vi "Process.vi"(8 "error in (no error)":errorcluster, 10 "pound in":refnum<class "Pound.lvclass">, 11 "qbus in":refnum<class "Qbus.lvclass">) -> (0 "error out":errorcluster)   [LabVIEW 2017, in "TracePointSynchronizer.lvlib"]
doc: "This process runs in the Server Comm module to send tracepoint instances to NI InsightCM Server and inform the Tracelogger process when the list of enabled tracepoints changes."
uses:
  <vilib>/addons/InsightCM/Devices/Shared/Common/TracePointSynchronizer/TracePointSynchronizer.lvlib
  <vilib>/addons/Qbus/Qbus.lvclass
  <vilib>/NI/Software Watchdog/Pound/Pound.lvclass
  <vilib>/addons/InsightCM/Devices/Shared/Common/TracePointSynchronizer/controls/config.ctl
  <vilib>/addons/InsightCM/Devices/Shared/Common/ServerComm/controls/ConnectionStatus.ctl
  <vilib>/addons/InsightCM/MessageBus/Base/controls/Message.ctl
  <vilib>/addons/InsightCM/MessageBus/Base/controls/MessageHeader.ctl
  <vilib>/addons/InsightCM/MessageBus/Base/controls/KeyValuePair.ctl
  <vilib>/addons/TimerProcess/controls/taskType.ctl
  <vilib>/addons/InsightCM/MessageBus/MessageLibrary/TraceLogger/controls/TraceLoggerCommandRequestBody.ctl
  <vilib>/addons/TraceLogger/controls/TracepointConfig.ctl
  <vilib>/addons/TraceLogger/TraceLogger.lvlib
  <vilib>/NI/Software Watchdog/Watchdog/Watchdog.lvclass
  <vilib>/addons/InsightCM/Devices/Shared/Common/ServerComm/ServerComm.lvlib
  <vilib>/addons/InsightCM/Utilities/GlobalConfiguration/GlobalConfiguration.lvlib
  <vilib>/addons/TimerProcess/TimerProcess.lvlib
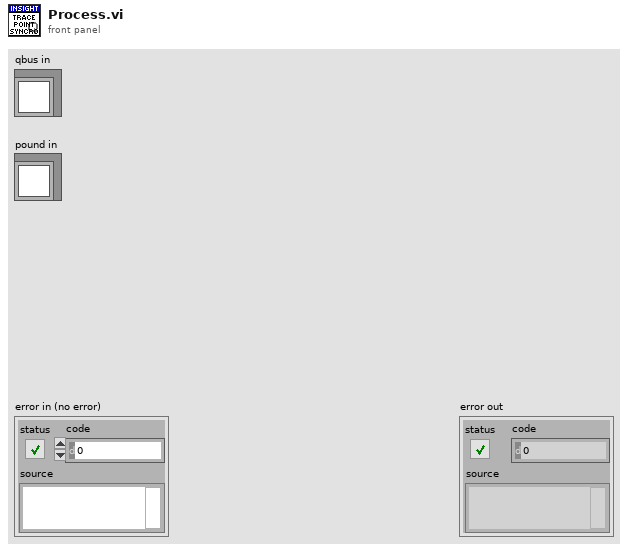
[diagram p1: front panel]
types:
  T1 = typedef "TracePointSynchronizer.lvlib/config.ctl" = cluster{"connection status":T2, "device name":string, "backlog messages":T3[], "log dir":path}
  T2 = typedef "ServerComm.lvlib/ConnectionStatus.ctl" = enum16{"Offline", "NotAuthorized", "Online"}
  T3 = typedef "Message.ctl" = cluster{"Header":T4, "Body":u8[]}
  T4 = typedef "MessageHeader.ctl" = cluster{"MessageName":string, "Timestamp":i64, "CorrelationId":string, "ContentType":string, "RoutingKey":string, "Properties":T5[]}
  T5 = typedef "KeyValuePair.ctl" = cluster{"Key":string, "Value":string}
  T6 = typedef "TimerProcess.lvlib/taskType.ctl" = enum16{"single", "repeat"}
  T7 = typedef "TraceLoggerCommandRequestBody.ctl" = cluster{"Arguments":string[]}
  T8 = typedef "TraceLogger.lvlib/TracepointConfig.ctl" = cluster{"name":string, "enabled":bool}
  T9 = typedef "R2_Device.ctl" = cluster{"Id":string, "Name":string, "DeviceType":string, "HardwareName":string, "IpAddress":string, "HardwareInfo":T5[], "ApplicationType":string, "ApplicationVersion":string, "EquipmentIds":string[], "ConfigurationVersion":string, "State":T10, "Properties":T5[], "DataGroups":T11[], "BurstModeTrigger":T15, "SensorGroups":T16[], "Endpoints":T17[]}
  T10 = typedef "DeviceState.ctl" = cluster{"Disabled":bool}
  T11 = typedef "R2_DataGroup.ctl" = cluster{"Name":string, "OperatingStates":T12[], "Properties":T5[], "EquipmentIds":string[], "AssetNodeId":string}
  T12 = typedef "OperatingState.ctl" = cluster{"Name":string, "Properties":T5[], "Triggers":T13[]}
  T13 = typedef "Trigger.ctl" = cluster{"Type":string, "Expression":string, "Conditions":T14[]}
  T14 = typedef "Condition.ctl" = cluster{"Source":string, "Type":string, "Operator":string, "CompareTo":string, "DwellSeconds":dbl}
  T15 = typedef "BurstModeTrigger.ctl" = cluster{"Trigger":T13, "SampleRate":string, "AcquisitionLength":string}
  T16 = typedef "DeviceSensorGroup.ctl" = cluster{"EquipId":string, "SensorGroupId":string}
  T17 = typedef "WirelessEndpoint.ctl" = cluster{"SerialNumber":string, "Properties":T5[], "Channels":T18[]}
  T18 = typedef "WirelessChannel.ctl" = cluster{"ChannelNumber":i32, "AssetId":string}
  T19 = typedef "TraceLoggerSnapshotBroadcastBody.ctl" = cluster{"Settings":T20[]}
  T20 = typedef "TracePointSetting.ctl" = cluster{"Name":string, "Enabled":bool, "Exceptions":string[]}
  T21 = typedef "TraceLogger.lvlib/LogTracepoint.ctl" = cluster{"tracepoint":string, "log string":string}
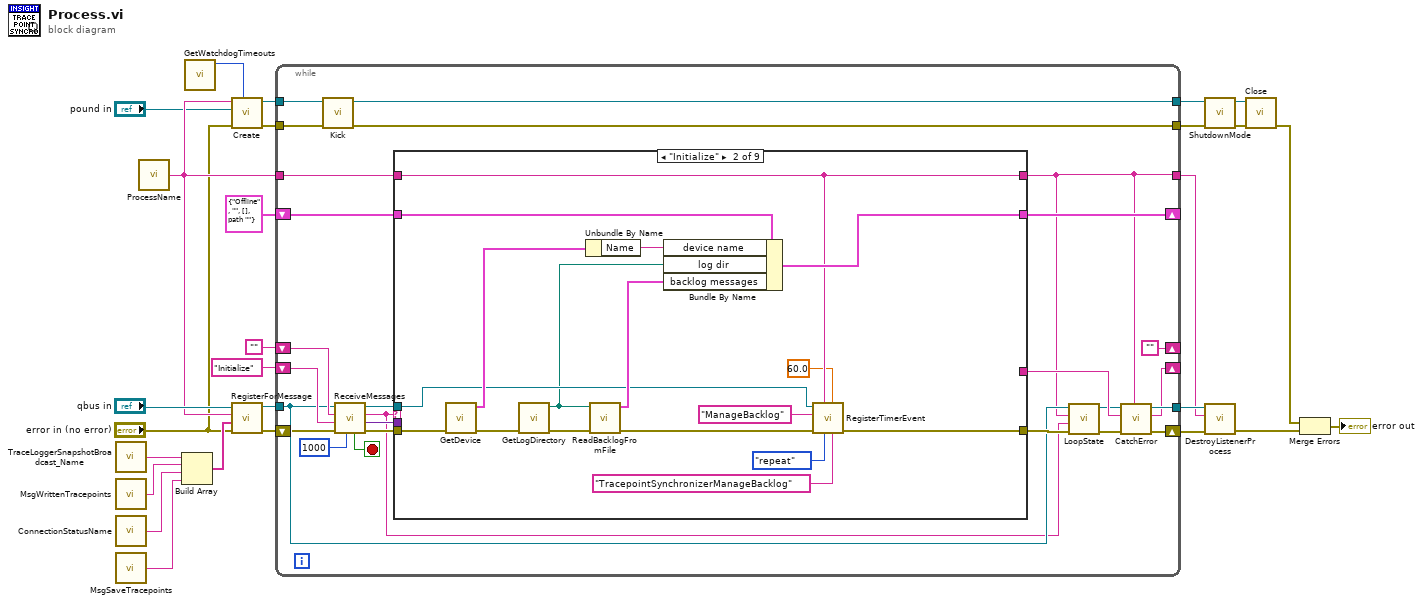
[diagram p0: block diagram]
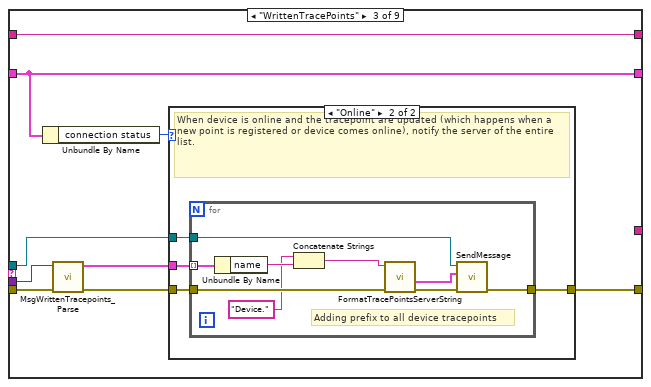
[diagram p3: hidden frame]
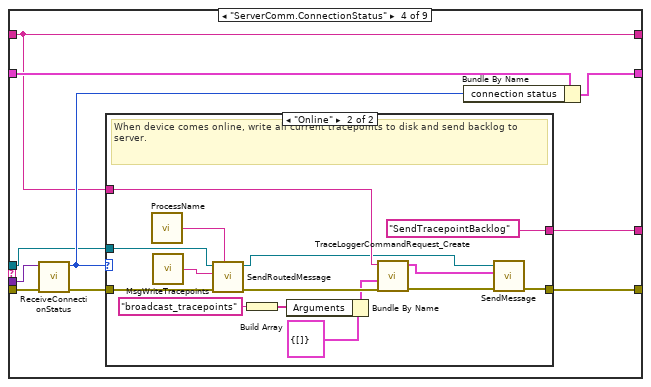
[diagram p5: hidden frame]
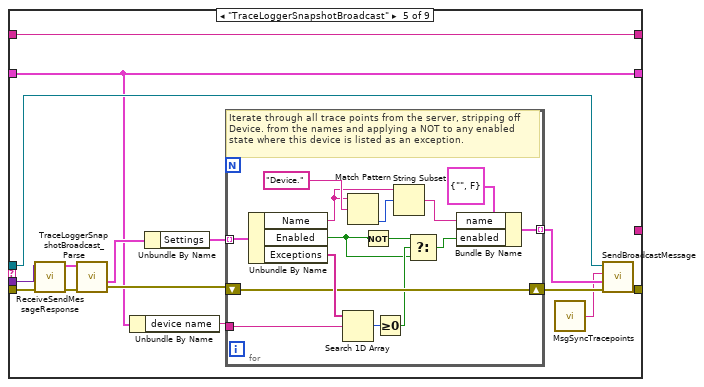
[diagram p7: hidden frame]
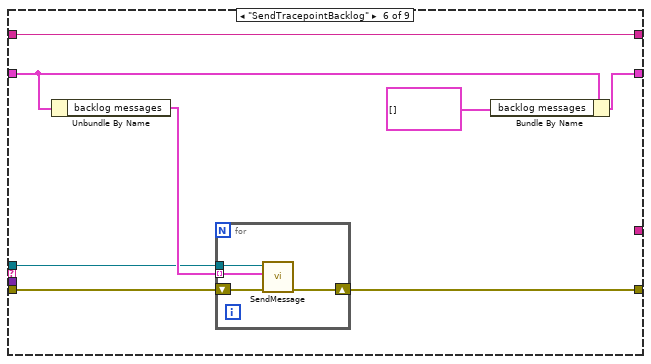
[diagram p8: hidden frame]
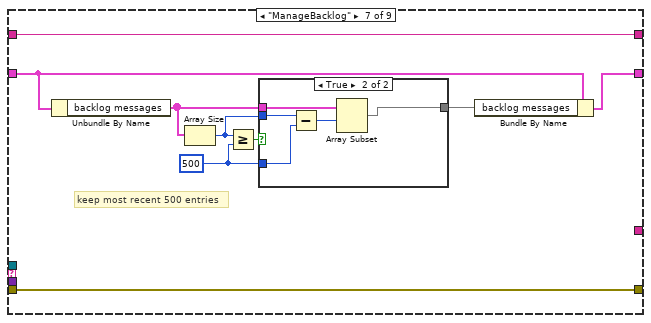
[diagram p9: hidden frame]
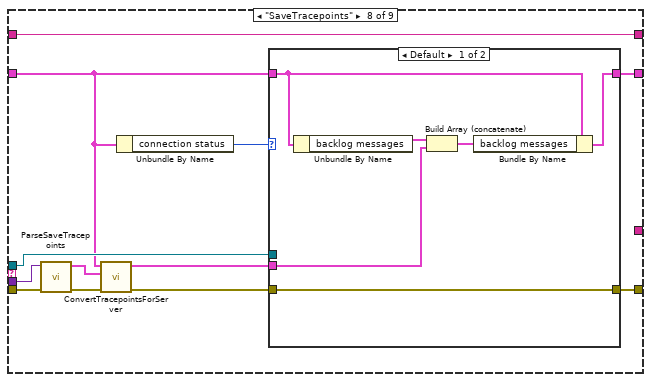
[diagram p11: hidden frame]
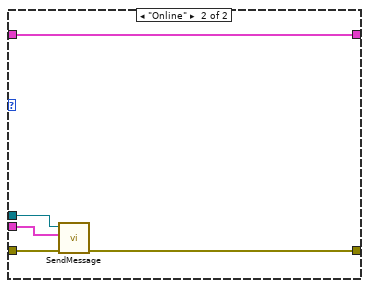
[diagram p12: hidden frame]
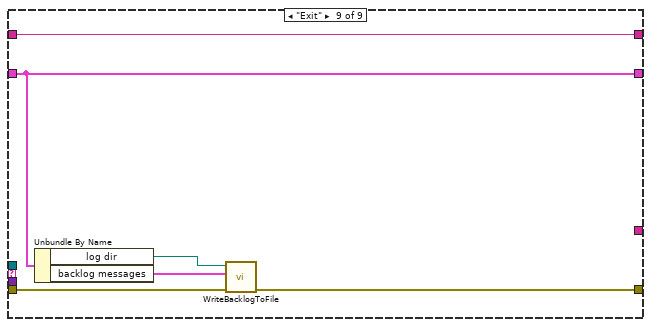
[diagram p13: hidden frame]
diagram:
  n1 = call <vilib>:"TraceLoggerSnapshotBroadcast_Name.vi"() -> ("MessageName"=w5:string)  [unwired: 5 in]
  n2 = call <vilib>:"MsgWrittenTracepoints.vi"() -> ("message name"=w4:string)  [unwired: 5 in]
  n3 = call <vilib>:"ConnectionStatusName.vi"() -> ("message name"=w3:string)  [unwired: 5 in]
  n4 = call <vilib>:"MsgSaveTracepoints.vi"() -> ("message name"=w2:string)  [unwired: 5 in]
  n5 = call <vilib>:"ProcessName.vi"() -> ("ProcessName"=w17:string)  [unwired: 5 in]
  n6 = Build Array(w5, w4, w3, w2) -> (w18:string[])
  n7 = call <vilib>:"GetWatchdogTimeouts.vi"() -> ("software timeout"=w1:u32)  [unwired: 10 in, 1 out]
  n8 = call <vilib>:"Create.vi"("Execution Timeout (ms)"=w1, "error in (no error)"="error in (no error)", "Pound"="pound in", "Name"=w17) -> ("error out"=w11:errorcluster, "Watchdog"=w16:refnum<data-value>)  [unwired: 6 in]
  n9 = call <vilib>:"RegisterForMessage.vi"("error in (no error)"="error in (no error)", "message names"=w18, "process name"=w17, "Qbus in"="qbus in") -> ("error in (no error)"=w26:errorcluster, "Qbus out"=w25:refnum<class "Qbus.lvclass">)  [unwired: 6 in]
  n10 = while {
    shift-right: [""] -> _
    shift-left: "" -> [w52]
    tunnel: w25 -> [w39]
    tunnel: w17 -> [w40]
    tunnel: [w43] -> w23
    tunnel: [w30] -> w22
    shift-right: [w42] -> _
    shift-left: "Initialize" -> [w47]
    shift-right: [w45] -> _
    shift-left: T1 {"connection status"=enum."Offline", "device name"="", "backlog messages"=[], "log dir"=path ""} ("config") -> [w46]
    tunnel: w16 -> [w38]
    tunnel: [w37] -> w13
    tunnel: w11 -> [w36]
    tunnel: [w34] -> w10
    shift-right: [w44] -> w24
    shift-left: w26 -> [w35]
    stop <- w53 stop-if-true
    n11 = call <vilib>:"Kick.vi"("error in (no error)"=w36, "Watchdog"=w38) -> ("error out"=w34:errorcluster, "Watchdog"=w37:refnum<data-value>)  [unwired: 8 in]
    n12 = call <vilib>:"ReceiveMessages.vi"("timeout(1000)"=1000 ("timeout(100)"), "error in (no error)"=w35, "priority action"=w47, "default action"=w52, "qbus in"=w39) -> ("error out"=w51:errorcluster, "message value"=w48:variant, "action"=w33:string, "qbus out"=w49:refnum<class "Qbus.lvclass">, "exit"=w53:bool)  [unwired: 2 in]
    n13 = case shown="\"Initialize\"" w33 {
      tunnel: w51 -> [w56 w73 w82 w106 w130 w156 w171 w191 w207]
      tunnel: w49 -> [_ w61 w79 w99 w133 w157 _ w187 _]
      tunnel: [w56 w60 w78 w101 w135 w155 w171 w186 w206] -> w41
      tunnel: w48 -> [_ _ w81 w105 w131 _ _ w190 _]
      tunnel: w46 -> [w55 w70 w80 w104 w125 w160 w173 w182 w208]
      tunnel: [w55 w69 w80 w103 w125 w159 w172 w181 w208] -> w45
      tunnel: w40 -> [w54 w63 w75 w97 w123 w153 w165 w180 w203]
      tunnel: [_ _ _ w98 _ _ _ _ _] -> w32
      tunnel: [w54 w63 w75 w97 w123 w153 w165 w180 w203] -> w30
      frame "", Default {
      }
      frame "Initialize" {
        n14 = call <vilib>:"GetDevice.vi"("error in (no error)"=w73) -> ("error out"=w59:errorcluster, "device configuration"=w72:T9)  [unwired: 8 in, 1 out]
        n15 = call <vilib>:"GetLogDirectory.vi"("error in (no error)"=w59) -> ("error out"=w58:errorcluster, "log dir"=w57:path)  [unwired: 9 in]
        n16 = Unbundle By Name(w72) -> ("Name"=w71:string)
        n17 = call <vilib>:"ReadBacklogFromFile.vi"("error in (no error)"=w58, "log dir"=w57) -> ("error out"=w64:errorcluster, "backlog messages"=w68:T3[])  [unwired: 8 in]
        n18 = Bundle By Name(cluster=w70, "device name"=w71, "log dir"=w57, "backlog messages"=w68) -> (w69:T1)
        n19 = call <vilib>:"RegisterTimerEvent.vi"("timer task name"="TracepointSynchronizerManageBacklog" ("Name"), "interval (sec)"=60.0, "type"=taskType."repeat", "process name"=w63, "error in (no error)"=w64, "callback action"="ManageBacklog", "qbus in"=w61) -> ("error out"=w60:errorcluster)  [unwired: 3 in, 1 out]
      }
      frame "WrittenTracePoints" {
        n20 = Unbundle By Name(w80) -> ("connection status"=w74:T2)
        n21 = call <vilib>:"MsgWrittenTracepoints_Parse.vi"("error in (no error)"=w82, "message body"=w81) -> ("error out"=w77:errorcluster, "data"=w76:T8[])  [unwired: 8 in]
        n22 = case shown="\"Online\"" w74 {
          tunnel: w79 -> [_ w87]
          tunnel: [w83 w86] -> w78
          tunnel: w77 -> [w83 w85]
          tunnel: w76 -> [_ w84]
          frame "Offline", Default {
          }
          frame "Online" {
            # "When device is online and the tracepoint are updated (which happens when a new point is registered or device comes online), notify the server of the entire list."
            n23 = for {
              tunnel: w87 -> [w94]
              tunnel: [w93] -> w86
              tunnel: w85 -> [w92]
              tunnel: w84 -> [w91] mode=indexing
              # "Adding prefix to all device tracepoints"
              n24 = Unbundle By Name(w91) -> ("name"=w90:string)
              n25 = Concatenate Strings("Device.", w90) -> (w89:string)
              n26 = call <vilib>:"FormatTracePointsServerString.vi"("error in"=w92, "TracePointName"=w89) -> ("error out"=w96:errorcluster, "Message out"=w95:T3)  [unwired: 8 in]
              n27 = call <vilib>:"SendMessage.vi"("error in (no error)"=w96, "message"=w95, "Qbus in"=w94) -> ("error out"=w93:errorcluster)  [unwired: 7 in, 1 out]
            }
          }
        }
      }
      frame "ServerComm.ConnectionStatus" {
        n28 = call <vilib>:"ReceiveConnectionStatus.vi"("error in (no error)"=w106, "body"=w105) -> ("error out"=w100:errorcluster, "status"=w102:T2)  [unwired: 6 in, 2 out]
        n29 = case shown="\"Online\"" w102 {
          tunnel: [w107 w110] -> w101
          tunnel: w100 -> [w107 w122]
          tunnel: w99 -> [_ w121]
          tunnel: [_ "SendTracepointBacklog"] -> w98
          tunnel: w97 -> [_ w116]
          frame Default {
          }
          frame "Online" {
            # "When device comes online, write all current tracepoints to disk and send backlog to server."
            n30 = call <vilib>:"ProcessName.vi"() -> ("process name"=w119:string)  [unwired: 5 in]
            n31 = call <vilib>:"MsgWriteTracepoints.vi"() -> ("message name"=w120:string)  [unwired: 5 in]
            n32 = call <vilib>:"SendRoutedMessage.vi"("listener process"=w119, "error in (no error)"=w122, "message name"=w120, "Qbus in"=w121) -> ("error in (no error)"=w117:errorcluster, "Qbus out"=w108:refnum<class "Qbus.lvclass">)  [unwired: 6 in]
            n33 = Build Array("broadcast_tracepoints") -> (w112:string[])
            n34 = Bundle By Name(cluster=T7 {"Arguments"=[]} ("TraceLoggerCommandRequest"), "Arguments"=w112) -> (w114:T7)
            n35 = call <vilib>:"TraceLoggerCommandRequest_Create.vi"("error in (no error)"=w117, "TraceLoggerCommandRequest"=w114, "ReplyTo"=w116) -> ("error out"=w111:errorcluster, "Message"=w109:T3)  [unwired: 7 in]
            n36 = call <vilib>:"SendMessage.vi"("error in (no error)"=w111, "message"=w109, "Qbus in"=w108) -> ("error out"=w110:errorcluster)  [unwired: 7 in, 1 out]
          }
        }
        n37 = Bundle By Name(cluster=w104, "connection status"=w102) -> (w103:T1)
      }
      frame "TraceLoggerSnapshotBroadcast" {
        n38 = call <vilib>:"ReceiveSendMessageResponse.vi"("error in (no error)"=w130, "body"=w131) -> ("error out"=w129:errorcluster, "message"=w128:T3)  [unwired: 6 in, 2 out]
        n39 = call <vilib>:"TraceLoggerSnapshotBroadcast_Parse.vi"("error in (no error)"=w129, "Message"=w128) -> ("error out"=w126:errorcluster, "Body"=w127:T19)  [unwired: 6 in, 2 out]
        n40 = Unbundle By Name(w125) -> ("device name"=w137:string)
        n41 = Unbundle By Name(w127) -> ("Settings"=w136:T20[])
        n42 = for {
          tunnel: w136 -> [w152] mode=indexing
          tunnel: w137 -> [w150]
          tunnel: [w147] -> w132 mode=indexing
          shift-right: [w146] -> w134
          shift-left: w126 -> [w146]
          # "Iterate through all trace points from the server, stripping off Device. from the names and applying a NOT to any enabled state where this device is listed as an exception."
          n43 = Unbundle By Name(w152) -> ("Name"=w139:string, "Enabled"=w142:bool, "Exceptions"=w151:string[])
          n44 = Search 1D Array(1D array=w151, element=w150) -> (index of element=w149:i32)  [unwired: 1 in]
          n45 = Match Pattern(string=w139, regular expression="Device.") -> (offset past match=w140:i32)  [unwired: 1 in, 3 out]
          n46 = Not(x=w142) -> (.not. x?=w143:bool)
          n47 = Greater Or Equal To 0?(x=w149) -> (x >= 0?=w145:bool)
          n48 = String Subset(string=w139, offset (0)=w140) -> (substring=w138:string)  [unwired: 1 in]
          n49 = Select(t=w143, s=w145, f=w142) -> (s? t:f=w144:bool)
          n50 = Bundle By Name(cluster=T8 {"name"="", "enabled"=FALSE} ("TracePoint"), "name"=w138, "enabled"=w144) -> (w147:T8)
        }
        n51 = call <vilib>:"MsgSyncTracepoints.vi"() -> ("message name"=w124:string)  [unwired: 5 in]
        n52 = call <vilib>:"SendBroadcastMessage.vi"("error in (no error)"=w134, "message value"=w132, "message name"=w124, "Qbus in"=w133) -> ("error in (no error)"=w135:errorcluster)  [unwired: 6 in, 1 out]
      }
      frame "SendTracepointBacklog" {
        n53 = Unbundle By Name(w160) -> ("backlog messages"=w158:T3[])
        n54 = for {
          tunnel: w158 -> [w164] mode=indexing
          tunnel: w157 -> [w163]
          shift-right: [w161] -> w155
          shift-left: w156 -> [w162]
          n55 = call <vilib>:"SendMessage.vi"("error in (no error)"=w162, "message"=w164, "Qbus in"=w163) -> ("error out"=w161:errorcluster)  [unwired: 7 in, 1 out]
        }
        n56 = Bundle By Name(cluster=w160, "backlog messages"=T3[] [] ("Backlog Messages")) -> (w159:T1)
      }
      frame "ManageBacklog" {
        w167 = 500
        # "keep most recent 500 entries"
        n57 = Unbundle By Name(w173) -> ("backlog messages"=w170:T3[])
        n58 = Array Size(array=w170) -> (size(s)=w168:i32)
        n59 = Greater Or Equal?(x=w168, y=w167) -> (x >= y?=w169:bool)
        n60 = case shown="True" w169 {
          tunnel: w170 -> [w174 w179]
          tunnel: w168 -> [_ w178]
          tunnel: w167 -> [_ w177]
          tunnel: [w174 w176] -> w166
          frame False {
          }
          frame True {
            n61 = Subtract(x=w178, y=w177) -> (x-y=w175:i32)
            n62 = Array Subset(array=w179, index=w175) -> (w176:T3[])  [unwired: 1 in]
          }
        }
        n63 = Bundle By Name(cluster=w173, "backlog messages"=w166) -> (w172:T1)
      }
      frame "SaveTracepoints" {
        n64 = call <vilib>:"ParseSaveTracepoints.vi"("error in (no error)"=w191, "message body"=w190) -> ("error out"=w188:errorcluster, "tracepoints"=w189:T21[])  [unwired: 8 in]
        n65 = call <vilib>:"ConvertTracepointsForServer.vi"("error in (no error)"=w188, "tracepoints"=w189, "config"=w182) -> ("error out"=w185:errorcluster, "message"=w184:T3)  [unwired: 7 in]
        n66 = Unbundle By Name(w182) -> ("connection status"=w183:T2)
        n67 = case shown="Default" w183 {
          tunnel: w187 -> [_ w202]
          tunnel: [w192 w201] -> w186
          tunnel: w185 -> [w192 w200]
          tunnel: w184 -> [w196 w199]
          tunnel: w182 -> [w195 w198]
          tunnel: [w193 w198] -> w181
          frame Default {
            n68 = Unbundle By Name(w195) -> ("backlog messages"=w197:T3[])
            n69 = Build Array (concatenate)(w197, w196) -> (w194:T3[])
            n70 = Bundle By Name(cluster=w195, "backlog messages"=w194) -> (w193:T1)
          }
          frame "Online" {
            n71 = call <vilib>:"SendMessage.vi"("error in (no error)"=w200, "message"=w199, "Qbus in"=w202) -> ("error out"=w201:errorcluster)  [unwired: 7 in, 1 out]
          }
        }
      }
      frame "Exit" {
        n72 = Unbundle By Name(w208) -> ("log dir"=w205:path, "backlog messages"=w204:T3[])
        n73 = call <vilib>:"WriteBacklogToFile.vi"("error in (no error)"=w207, "backlog messages"=w204, "log dir"=w205) -> ("error out"=w206:errorcluster)  [unwired: 8 in]
      }
    }
    n74 = call <vilib>:"LoopState.vi"("error in (no error)"=w41, "loop action"=w33, "process name"=w30, "Qbus in"=w39) -> ("error out"=w29:errorcluster, "Qbus out"=w28:refnum<class "Qbus.lvclass">)  [unwired: 6 in]
    n75 = call <vilib>:"CatchError.vi"("source"=w30, "error in (no error)"=w29, "next action in"=w32, "Qbus in"=w28) -> ("error out"=w44:errorcluster, "next action out"=w42:string, "Qbus out"=w43:refnum<class "Qbus.lvclass">)  [unwired: 5 in]
  }
  n76 = call <vilib>:"ShutdownMode.vi"("error in (no error)"=w10, "Watchdog"=w13) -> ("error out"=w12:errorcluster, "Watchdog"=w14:refnum<data-value>)  [unwired: 8 in]
  n77 = call <vilib>:"DestroyListenerProcess.vi"("error in (no error)"=w24, "process name"=w22, "Qbus in"=w23) -> ("error in (no error)"=w9:errorcluster)  [unwired: 7 in, 1 out]
  n78 = call <vilib>:"Close.vi"("error in (no error)"=w12, "Watchdog"=w14) -> ("error out"=w8:errorcluster)  [unwired: 9 in]
  n79 = Merge Errors(w8, w9) -> (→"error out":errorcluster)
